vi "读取bool_ref.vi"(8 "error in (no error)":errorcluster caption="错误输入（无错误）", 11 "RandomMoveBool输入":refnum<class "RandomMoveBool.lvclass">) -> (0 "error out":errorcluster caption="错误输出", 2 "bool_ref":refnum<vi>, 3 "RandomMoveBool输出":refnum<class "RandomMoveBool.lvclass">)   [LabVIEW 2018, in "RandomMoveBool.lvclass"]
uses:
  RandomMoveBool.lvclass
  RandomMoveBool.lvclass/RandomMoveBool.ctl
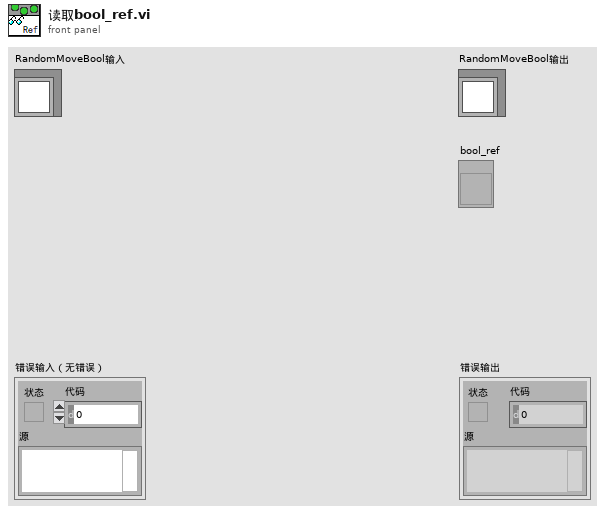
[diagram p1: front panel]
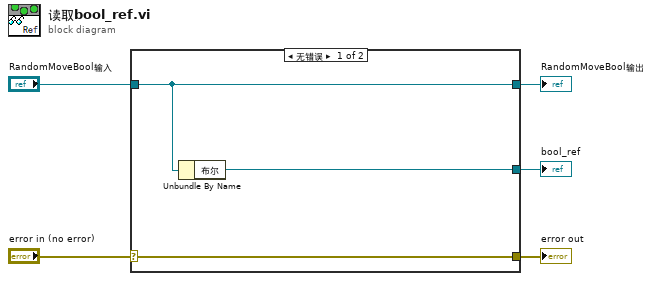
[diagram p0: block diagram]
diagram:
  n1 = case shown="无错误" "error in (no error)" {
    selector: "error in (no error)" -> [w8 w9]
    tunnel: [w8 w9] -> w4
    tunnel: [w7 w10] -> w2
    tunnel: "RandomMoveBool输入" -> [w7 w10]
    tunnel: [w6 _] -> w1
    frame No Error {
      n2 = Unbundle By Name(w7) -> ("布尔"=w6:refnum<vi>)
    }
    frame Error {
    }
  }
  "error out" <- w4
  "RandomMoveBool输出" <- w2
  "bool_ref" <- w1
